vi "ConfigSetterTemplate.vi"(6 "timeoutSeconds":dbl, 8 "FutureProofConfigs":bool, 10 "Configs":string, 11 "DeviceReference":T1) -> (3 "StatusCode":i32)   [LabVIEW 2023]
uses:
  Users/Cory/Documents/PhoenixPro-LabVIEW-Generation/controls/DeviceReference.ctl
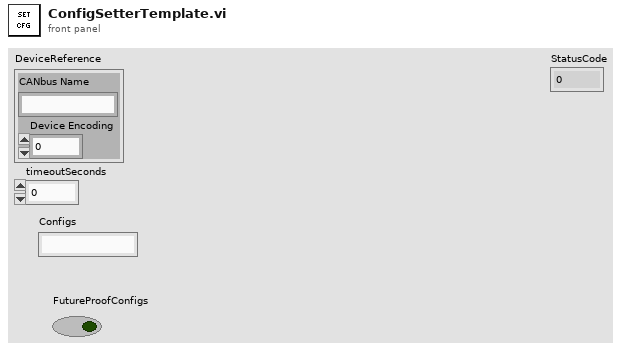
[diagram p1: front panel]
types:
  T1 = typedef "DeviceReference.ctl" = cluster{"CANbus Name":string, "Device Encoding":u32}
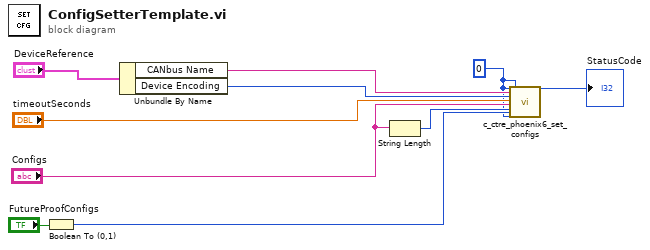
[diagram p0: block diagram]
diagram:
  w2 = 0 ("Numeric 2")
  n1 = Boolean To (0,1)(Boolean="FutureProofConfigs") -> (0, 1=w3:i16)
  n2 = Unbundle By Name("DeviceReference") -> ("CANbus Name"=w9:string, "Device Encoding"=w8:u32)
  n3 = String Length(string="Configs") -> (length=w5:i32)
  n4 = call <vilib>:"c_ctre_phoenix6_set_configs.vi"("Numeric 2"=w2, "String 2"=w9, "Numeric 3"=w8, "Numeric 4"="timeoutSeconds", "String 4"="Configs", "Numeric 5"=w5, "Numeric 6"=w3, "Numeric 7"=w2, "Numeric 8"=w2) -> ("Numeric"=→"StatusCode":i32)  [unwired: 16 in, 2 out]
